vi "Parse Positions and Speeds.vi"(11 "standard output":string) -> (2 "Array":dbl[](array[numeric]), 3 "Array 2":dbl[](array[numeric]))   [LabVIEW 2020, in "Manipulator CLI Driver.lvlib"]
uses:
  Manipulator CLI Driver.lvlib
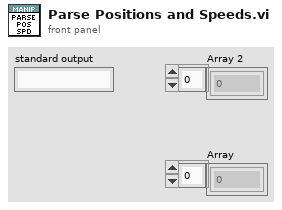
[diagram p1: front panel]
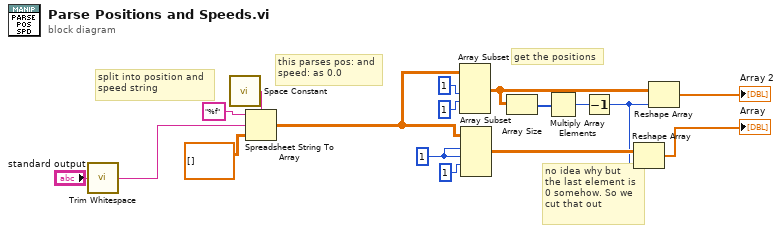
[diagram p0: block diagram]
diagram:
  w14 = 1 ("index")
  # "no idea why but\nthe last element is\n0 somehow. So we\ncut that out"
  # "get the positions"
  # "this parses pos: and\nspeed: as 0.0"
  # "split into position and\nspeed string"
  n1 = call <vilib>:"Trim Whitespace.vi"("string"="standard output") -> ("trimmed string"=w4:string)  [unwired: 1 in]
  n2 = call <vilib>:"Space Constant.vi"() -> ("String"=w6:string)
  n3 = Spreadsheet String To Array(delimiter (Tab)=w6, format string="%f", spreadsheet string=w4, array type (2D Dbl)=dbl[][] []) -> (array=w12:dbl[][])
  n4 = Array Subset(array=w12, length (row)=1 ("index"), index (col)=1 ("length")) -> (w15:dbl[][])  [unwired: 2 in]
  n5 = Array Subset(array=w12, index (row)=w14, length (row)=w14, index (col)=1 ("length")) -> (w11:dbl[][])  [unwired: 1 in]
  n6 = Array Size(array=w15) -> (size(s)=w16:i32[])
  n7 = Multiply Array Elements(1:w16) -> (0:w17:i32)
  n8 = Decrement(x=w17) -> (x-1=w1:i32)
  n9 = Reshape Array(w11, w1) -> (→"Array":dbl[])
  n10 = Reshape Array(w15, w1) -> (→"Array 2":dbl[])
